vi "Get Status Channels.vi"(8 "error in (no error)":errorcluster, 11 "Device Ref in":T1 format="%.0x") -> (0 "error out":errorcluster, 1 "Error Code Ref":T1 format="%.0x", 2 "Connection Status Ref":T1 format="%.0x", 3 "Device Ref out":T1 format="%.0x")   [LabVIEW 2012, in "Shared Variable Custom Device.lvlib"]
doc: "Get references for the Status channels."
uses:
  Shared Variable Custom Device.lvlib
  <vilib>/NI Veristand/Custom Device API/Custom Device Item Ref.ctl
  Shared/Shared Variable GUID Lookup.vi
  <vilib>/NI Veristand/Custom Device Tools/Custom Device Utility Library/NI VeriStand - Search for Item by GUID.vi
  <vilib>/NI Veristand/Custom Device Tools/Custom Device Utility Library/Custom Device Utility Library.lvlib
  <vilib>/NI Veristand/Custom Device API/Custom Device API.lvlib
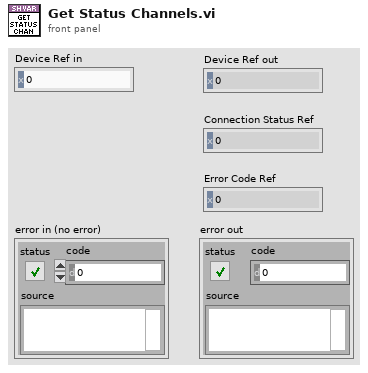
[diagram p1: front panel]
types:
  T1 = typedef "Custom Device API.lvlib/Custom Device Item Ref.ctl" = u64
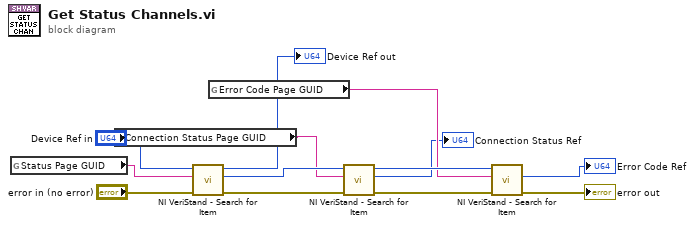
[diagram p0: block diagram]
diagram:
  n1 = global read "Shared Variable GUID Lookup.vi" "Status Page GUID"() -> (w8:string)
  n2 = global read "Shared Variable GUID Lookup.vi" "Connection Status Page GUID"() -> (w4:string)
  n3 = call-poly <vilib>:"NI VeriStand - Search for Item.vi"("error in"="error in (no error)", "Item GUID"=w8, "Section Ref in"="Device Ref in") -> ("error out"=w9:errorcluster, "Item Ref"=w10:T1, "Section Ref out"=→"Device Ref out":T1)  [unwired: 5 in, 1 out]
  n4 = global read "Shared Variable GUID Lookup.vi" "Error Code Page GUID"() -> (w3:string)
  n5 = call-poly <vilib>:"NI VeriStand - Search for Item.vi"("error in"=w9, "Item GUID"=w4, "Section Ref in"=w10) -> ("error out"=w5:errorcluster, "Item Ref"=→"Connection Status Ref":T1, "Section Ref out"=w6:T1)  [unwired: 5 in, 1 out]
  n6 = call-poly <vilib>:"NI VeriStand - Search for Item.vi"("error in"=w5, "Item GUID"=w3, "Section Ref in"=w6) -> ("error out"=→"error out":errorcluster, "Item Ref"=→"Error Code Ref":T1)  [unwired: 5 in, 2 out]
